vi "Two_Qubits_Swap.vi"(6 "ControlArray":bool[][](array[boolean]), 8 "error in (no error)":errorcluster, 9 "SwapingWiresIndex":i32[](array[numeric]), 10 "QuWire in":refnum<class "QuWire.lvclass">, 11 "SimAlg in":refnum<class "PrllPerElmnt.lvclass">) -> (0 "error out":errorcluster, 2 "QuWire out":refnum<class "QuWire.lvclass">, 3 "SimAlg out":refnum<class "PrllPerElmnt.lvclass">)   [LabVIEW 2020, in "PrllPerElmnt.lvclass"]
uses:
  PrllPerElmnt.lvclass
  QuWire/QuWire.lvclass
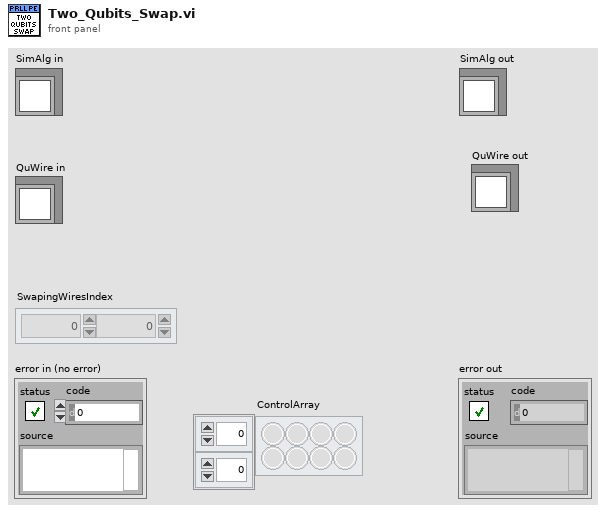
[diagram p1: front panel]
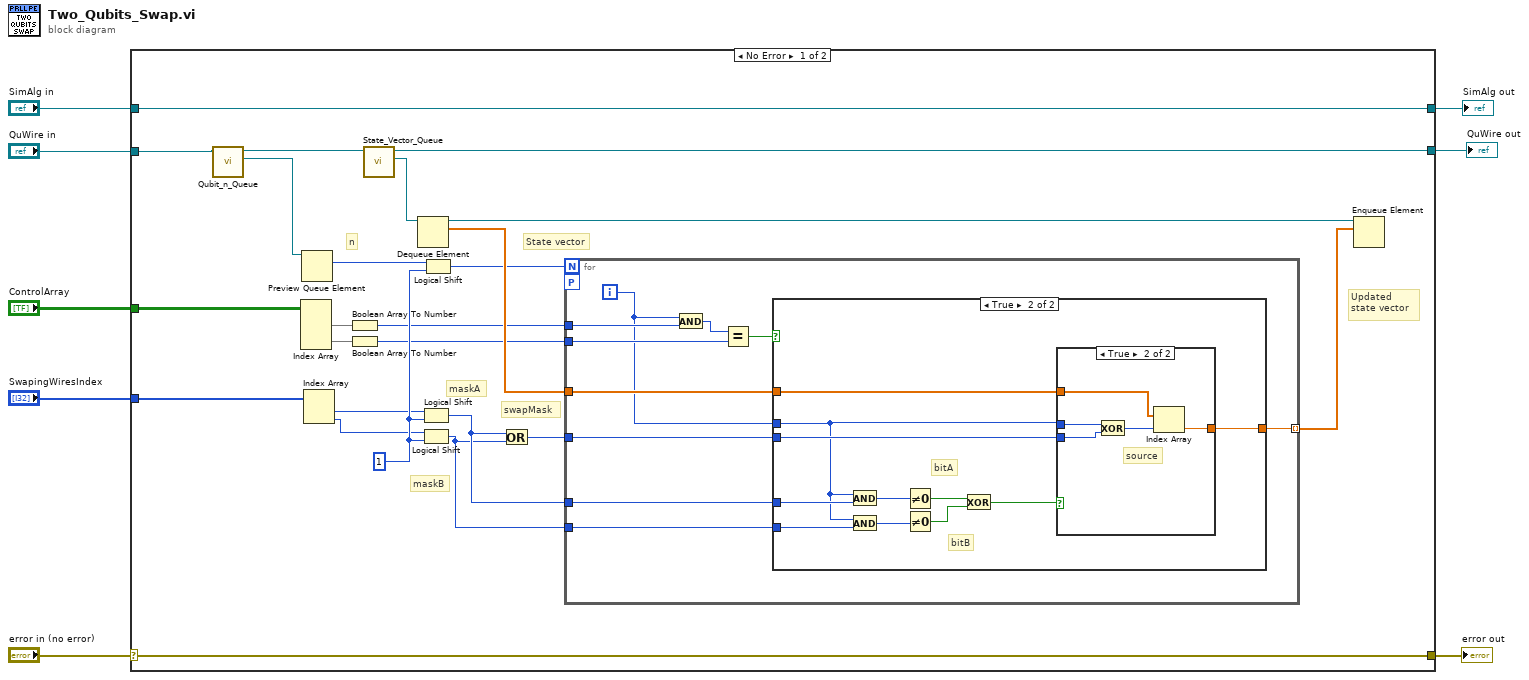
[diagram p0: block diagram]
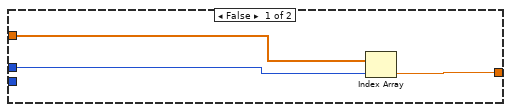
[diagram p2: hidden frame]
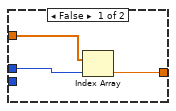
[diagram p3: hidden frame]
diagram:
  n1 = case shown="No Error" "error in (no error)" {
    selector: "error in (no error)" -> [w31 w67]
    tunnel: [w31 w67] -> w7
    tunnel: [w32 w66] -> w5
    tunnel: "SimAlg in" -> [w32 w66]
    tunnel: "QuWire in" -> [w12 w65]
    tunnel: [w11 w65] -> w3
    tunnel: "ControlArray" -> [w10 _]
    tunnel: "SwapingWiresIndex" -> [w9 _]
    frame No Error {
      w23 = 1 ("x")
      # "Updated state vector"
      # "swapMask"
      # "maskB"
      # "maskA"
      # "State vector"
      # "n"
      n2 = call "Qubit_n_Queue.vi"("QuWire in"=w12) -> ("Qubit n"=w25:refnum<queue>, "QuWire out"=w24:refnum<class "QuWire.lvclass">)  [unwired: 8 in, 1 out]
      n3 = Index Array(array=w10) -> (element #1=w13:bool[], element #2=w14:bool[])  [unwired: 4 in]
      n4 = Preview Queue Element(queue=w25) -> (element=w26:i32)  [unwired: 2 in, 3 out]
      n5 = Index Array(array=w9) -> (element #1=w19:i32, element #2=w22:i32)  [unwired: 2 in]
      n6 = Boolean Array To Number(Boolean array=w13) -> (number=w20:u32)
      n7 = Boolean Array To Number(Boolean array=w14) -> (number=w21:u32)
      n8 = call "State_Vector_Queue.vi"("QuWire in"=w24) -> ("State Vector Queue"=w27:refnum<queue>, "QuWire out"=w11:refnum<class "QuWire.lvclass">)  [unwired: 8 in, 1 out]
      n9 = Dequeue Element(queue=w27) -> (queue out=w29:refnum<queue>, element=w28:cdb[])  [unwired: 2 in, 2 out]
      n10 = Logical Shift(y=w19, x=w23) -> (x << y=w17:i32)
      n11 = Logical Shift(y=w22, x=w23) -> (x << y=w16:i32)
      n12 = Logical Shift(y=w26, x=w23) -> (x << y=w18:i32)
      n13 = Or(x=w17, y=w16) -> (x .or. y?=w15:i32)
      n14 = for {
        N: w18 -> [_]
        tunnel: w28 -> [w38]
        tunnel: w20 -> [w41]
        tunnel: w21 -> [w39]
        tunnel: [w33] -> w30 mode=indexing
        tunnel: w17 -> [w37]
        tunnel: w16 -> [w36]
        tunnel: w15 -> [w35]
        workers-P: _ -> [_]
        i -> [w34]
        n15 = And(x=w34, y=w41) -> (x .and. y?=w42:u32)
        n16 = Equal?(x=w42, y=w39) -> (x = y?=w40:bool)
        n17 = case shown="True" w40 {
          tunnel: w38 -> [w45 w48]
          tunnel: w37 -> [_ w53]
          tunnel: w36 -> [_ w52]
          tunnel: w35 -> [_ w49]
          tunnel: w34 -> [w43 w46]
          tunnel: [w44 w47] -> w33
          frame False {
            n18 = Index Array(array=w45, index=w43) -> (element=w44:cdb)
          }
          frame True {
            # "bitB"
            # "bitA"
            n19 = And(x=w46, y=w53) -> (x .and. y?=w55:i32)
            n20 = And(x=w46, y=w52) -> (x .and. y?=w56:i32)
            n21 = Not Equal To 0?(x=w55) -> (x != 0?=w51:bool)
            n22 = Not Equal To 0?(x=w56) -> (x != 0?=w54:bool)
            n23 = Exclusive Or(1:w54, 2:w51) -> (0:w50:bool)
            n24 = case shown="True" w50 {
              tunnel: w49 -> [_ w64]
              tunnel: w46 -> [w58 w63]
              tunnel: w48 -> [w59 w62]
              tunnel: [w57 w60] -> w47
              frame False {
                n25 = Index Array(array=w59, index=w58) -> (element=w57:cdb)
              }
              frame True {
                # "source"
                n26 = Exclusive Or(1:w64, 2:w63) -> (0:w61:i32)
                n27 = Index Array(array=w62, index=w61) -> (element=w60:cdb)
              }
            }
          }
        }
      }
      n28 = Enqueue Element(queue=w29, element=w30) -> ()  [unwired: 2 in, 3 out]
    }
    frame Error {
    }
  }
  "error out" <- w7
  "SimAlg out" <- w5
  "QuWire out" <- w3
